vi "Configure Hardware.vi"(8 "error in (no error)":errorcluster, 11 "Hardware Resources in":T1) -> (0 "error out":errorcluster, 3 "Hardware Resources out":T1)   [LabVIEW 2016, in "Acquisition.lvlib"]
doc: "Configure the hardware."
uses:
  Acquisition.lvlib
  Hardware Configuration.ctl
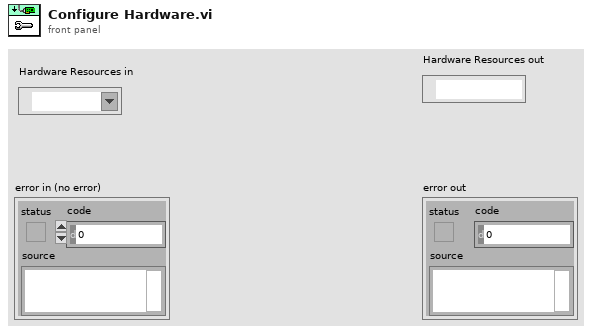
[diagram p1: front panel]
types:
  T1 = typedef "Acquisition.lvlib/Hardware Configuration.ctl" = refnum<visa-resource-name>
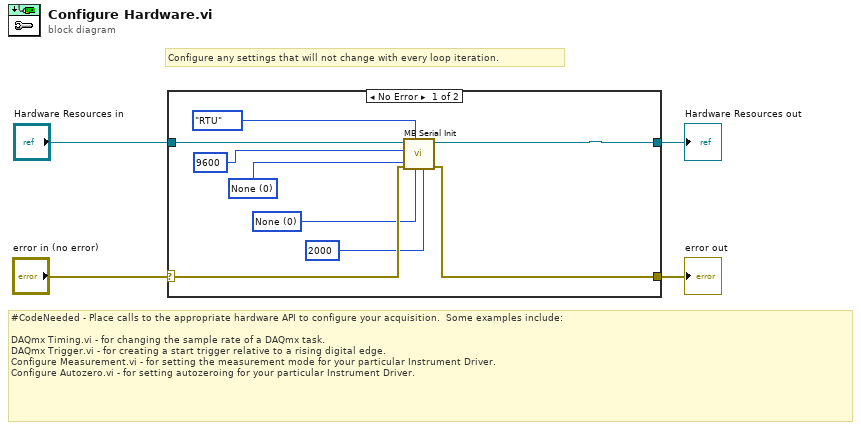
[diagram p0: block diagram]
diagram:
  # "Configure any settings that will not change with every loop iteration."
  # "#CodeNeeded - Place calls to the appropriate hardware API to configure your acquisition.  Some examples include:\n\nDAQmx Timing.vi - for changing the sample rate of a DAQmx task.\nDAQmx Trigger.vi - for creating a start trigger relative to a rising digital edge.\nConfigure Measurement.vi - for setting the measurement mode for your particular Instrument Driver.\nConfigure Autozero.vi - for setting autozeroing for your particular Instrument Driver."
  n1 = case shown="No Error" "error in (no error)" {
    selector: "error in (no error)" -> [w8 w14]
    tunnel: [w7 w14] -> w3
    tunnel: "Hardware Resources in" -> [w13 w15]
    tunnel: [w12 w15] -> w1
    frame No Error {
      w6 = u16 0 items=["None", "XON/XOFF", "RTS/CTS", "XON/XOFF & RTS/CTS", "DTR/DSR", "XON/XOFF & DTR/DSR"] ("Flow Control")
      w10 = u16 0 items=["None", "Odd", "Even", "Mark", "Space"] ("Parity")
      n2 = call <vilib>:"MB Serial Init.vi"("Timeout"=u32 2000, "Flow Control"=w6, "Mode"=enum16{"RTU", "ASCII"}."RTU", "error in (no error)"=w8, "Parity"=w10, "Baud Rate"=u32 9600, "VISA resource name"=w13) -> ("error out"=w7:errorcluster, "VISA resource name out"=w12:refnum<visa-resource-name>)  [unwired: 3 in]
    }
    frame Error {
    }
  }
  "Hardware Resources out" <- w1
  "error out" <- w3
